vi "CavityModelConstants.vi"(0 "w12":dbl format="%#_12g", 5 "R1":dbl, 7 "w1":dbl, 9 "Q1":dbl, 11 "K1":dbl, 12 "S":dbl) -> (4 "C1":dbl, 6 "C2":dbl, 8 "C3":dbl, 10 "C4":dbl, 15 "C5":dbl)   [LabVIEW 2013]
panel:
  # "w12, Rl, w1, Q1 och K1"
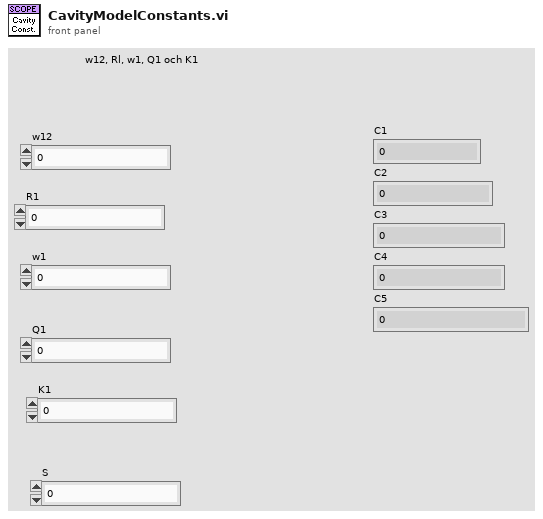
[diagram p1: front panel]
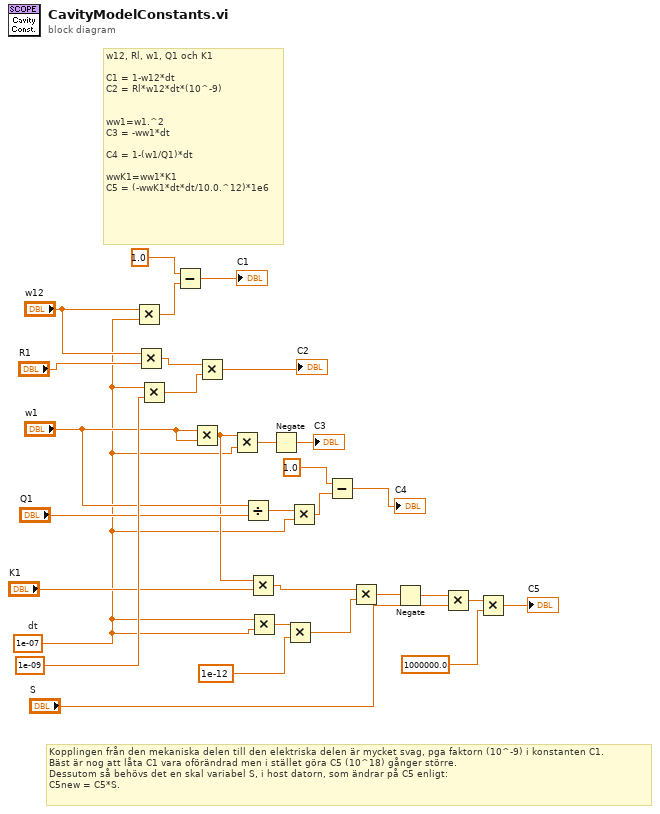
[diagram p0: block diagram]
diagram:
  w7 = 1e-07  # dt
  # "Kopplingen från den mekaniska delen till den elektriska delen är mycket svag, pga faktorn (10^-9) i konstanten C1.\nBäst är nog att låta C1 vara oförändrad men i stället göra C5 (10^18) gånger större.\nDessutom så behövs det en skal variabel S, i host datorn, som ändrar på C5 enligt: \nC5new = C5*S."
  # "w12, Rl, w1, Q1 och K1\n\nC1 = 1-w12*dt\nC2 = Rl*w12*dt*(10^-9)\n\n\nww1=w1.^2\nC3 = -ww1*dt\n\nC4 = 1-(w1/Q1)*dt\n\nwwK1=ww1*K1\nC5 = (-wwK1*dt*dt/10.0.^12)*1e6"
  n1 = Multiply(x="w12", y=w7) -> (x*y=w24:dbl)
  n2 = Multiply(x="w12", y="R1") -> (x*y=w28:dbl)
  n3 = Multiply(x=w7, y=1e-09) -> (x*y=w27:dbl)
  n4 = Subtract(x=1.0, y=w24) -> (x-y=→"C1":dbl)
  n5 = Multiply(x="w1", y="w1") -> (x*y=w18:dbl)
  n6 = Multiply(x=w28, y=w27) -> (x*y=→"C2":dbl)
  n7 = Multiply(x=w18, y=w7) -> (x*y=w23:dbl)
  n8 = Divide(x="w1", y="Q1") -> (x/y=w14:dbl)
  n9 = Multiply(x=w18, y="K1") -> (x*y=w16:dbl)
  n10 = Multiply(x=w7, y=w7) -> (x*y=w6:dbl)
  n11 = Negate(x=w23) -> (-x=→"C3":dbl)
  n12 = Multiply(x=w6, y=1e-12) -> (x*y=w4:dbl)
  n13 = Multiply(x=w14, y=w7) -> (x*y=w13:dbl)
  n14 = Subtract(x=1.0, y=w13) -> (x-y=→"C4":dbl)
  n15 = Multiply(x=w16, y=w4) -> (x*y=w15:dbl)
  n16 = Negate(x=w15) -> (-x=w9:dbl)
  n17 = Multiply(x=w9, y="S") -> (x*y=w3:dbl)
  n18 = Multiply(x=w3, y=1000000.0) -> (x*y=→"C5":dbl)
